vi "AG34980A_List_to_Array.vi"(4 "List":string, 7 "Separator (,)":string=",") -> (0 "Output Number Array":dbl[](array[numeric]) format="%.2f", 3 "Output String Array":string[](array[string]))   [LabVIEW 2022 SP3]
doc: "Given a List of strings separated by a Separator, this VI returns the List as a String Array. If the strings are numbers, a Number Array is also returned."
uses:
  <vilib>/Utility/error.llb/Trim Whitespace One-Sided.vi
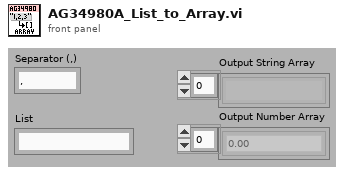
[diagram p1: front panel]
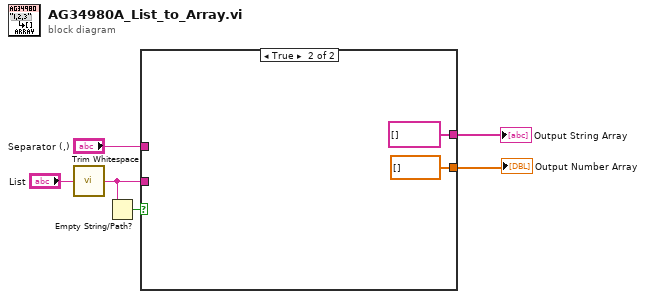
[diagram p0: block diagram]
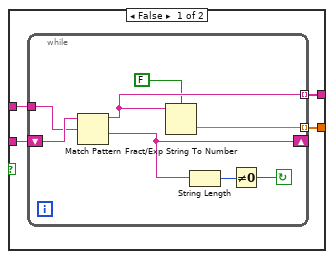
[diagram p2: hidden frame]
diagram:
  n1 = call <vilib>:"Trim Whitespace.vi"("string"="List") -> ("trimmed string"=w2:string)  [unwired: 1 in]
  n2 = Empty String/Path?(string/path=w2) -> (empty?=w1:bool)
  n3 = case shown="True" w1 {
    tunnel: "Separator (,)" -> [w10 _]
    tunnel: [w9 string[] []] -> w5
    tunnel: [w8 dbl[] []] -> w4
    tunnel: w2 -> [w7 _]
    frame False {
      n4 = while {
        tunnel: w10 -> [w12]
        tunnel: [w13] -> w9 mode=indexing
        tunnel: [w15] -> w8 mode=indexing
        shift-left: w7 -> [w16]
        shift-right: [w14] -> _
        stop <- w18 continue-if-true
        n5 = Match Pattern(string=w16, regular expression=w12) -> (before substring=w13:string, after substring=w14:string)  [unwired: 1 in, 2 out]
        n6 = Fract/Exp String To Number(use system decimal point (T)=FALSE, string=w13) -> (number=w15:dbl)  [unwired: 2 in, 1 out]
        n7 = String Length(string=w14) -> (length=w17:i32)
        n8 = Not Equal To 0?(x=w17) -> (x != 0?=w18:bool)
      }
    }
    frame True {
    }
  }
  "Output String Array" <- w5
  "Output Number Array" <- w4
